vi "build-scan-pts-list.vi"(10 "Y in":cluster{"start":dbl, "stop":dbl, "step":dbl}, 11 "X in":cluster{"start":dbl, "stop":dbl, "step":dbl}) -> (2 "Y out":dbl[](array[numeric]), 3 "X out":dbl[](array[numeric]))   [LabVIEW 2024]
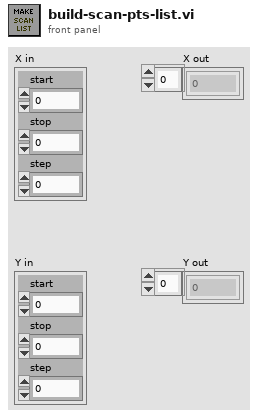
[diagram p1: front panel]
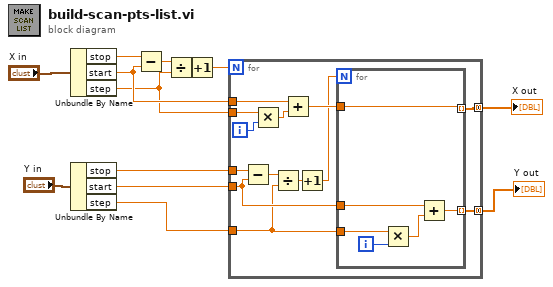
[diagram p0: block diagram]
diagram:
  n1 = Unbundle By Name("X in") -> ("stop"=w6:dbl, "start"=w5:dbl, "step"=w4:dbl)
  n2 = Unbundle By Name("Y in") -> ("stop"=w3:dbl, "start"=w2:dbl, "step"=w1:dbl)
  n3 = Subtract(x=w6, y=w5) -> (x-y=w9:dbl)
  n4 = Divide(x=w9, y=w4) -> (x/y=w8:dbl)
  n5 = Increment(x=w8) -> (x+1=w7:dbl)
  n6 = for {
    N: w7 -> [_]
    tunnel: w5 -> [w25]
    tunnel: [w22] -> w10 mode=concatenating
    tunnel: [w21] -> w11 mode=concatenating
    tunnel: w4 -> [w17]
    tunnel: w3 -> [w16]
    tunnel: w2 -> [w15]
    tunnel: w1 -> [w14]
    i -> [w26]
    n7 = Subtract(x=w16, y=w15) -> (x-y=w20:dbl)
    n8 = Multiply(x=w17, y=w26) -> (x*y=w24:dbl)
    n9 = Divide(x=w20, y=w14) -> (x/y=w19:dbl)
    n10 = Add(x=w25, y=w24) -> (x+y=w23:dbl)
    n11 = Increment(x=w19) -> (x+1=w18:dbl)
    n12 = for {
      N: w18 -> [_]
      tunnel: w23 -> [w32]
      tunnel: [w32] -> w22 mode=indexing
      tunnel: [w29] -> w21 mode=indexing
      tunnel: w15 -> [w28]
      tunnel: w14 -> [w27]
      i -> [w30]
      n13 = Multiply(x=w27, y=w30) -> (x*y=w31:dbl)
      n14 = Add(x=w28, y=w31) -> (x+y=w29:dbl)
    }
  }
  "Y out" <- w11
  "X out" <- w10
